vi "获取波形子集.vi"(1 "duration":dbl=1.0 caption="持续时间" format="%0.2f", 2 "start samples/time":dbl caption="起始采样/时间" format="%0.2f", 3 "时域波形图":waveform(dbl)[](graph)) -> (0 "时域波形图 2":waveform(dbl)[](graph))   [LabVIEW 2014]
uses:
  <vilib>/Waveform/WDTOps.llb/WDT Get Waveform Subset DBL.vi
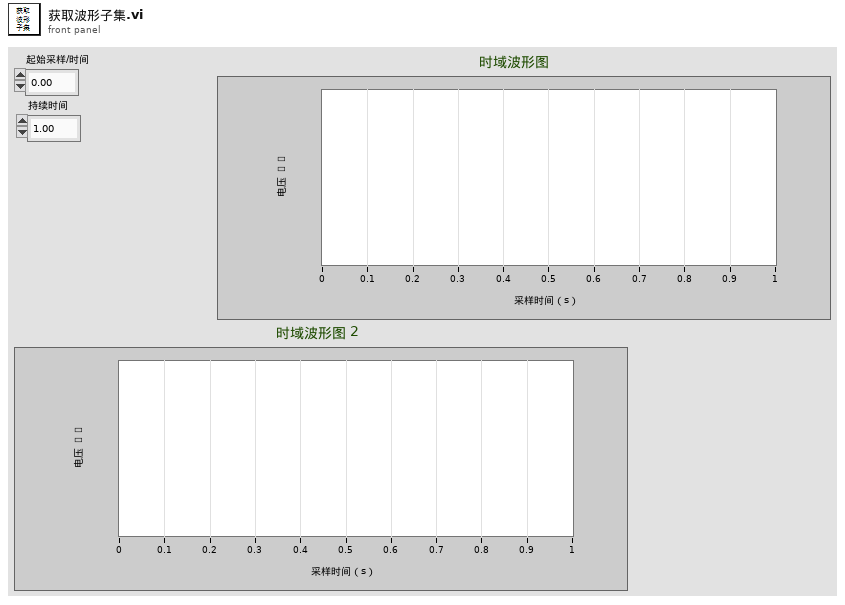
[diagram p1: front panel]
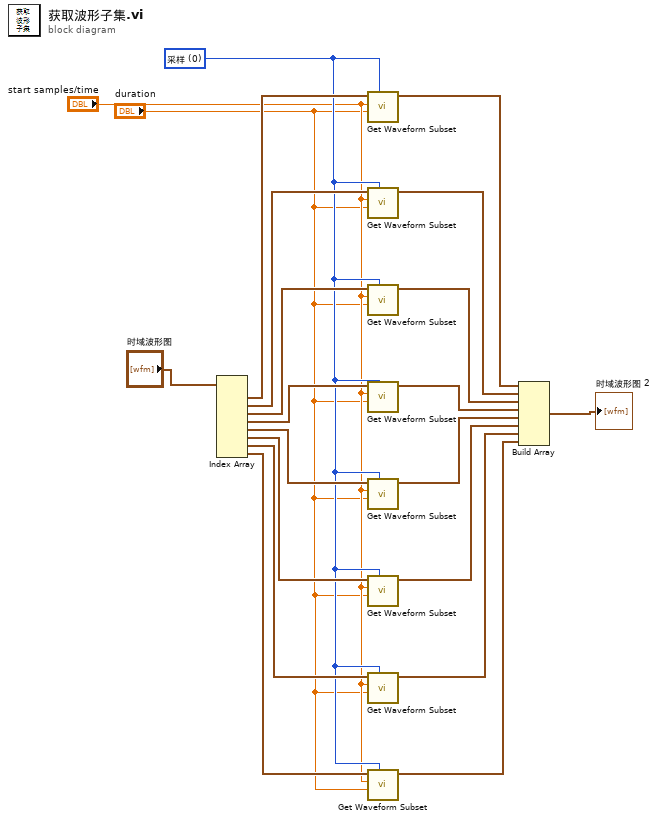
[diagram p0: block diagram]
diagram:
  w12 = u16 0 items=["采样", "相对时间"] ("start/duration format")
  n1 = Index Array(array="时域波形图") -> (element #1=w20:waveform(dbl), element #2=w19:waveform(dbl), element #3=w18:waveform(dbl), element #4=w17:waveform(dbl), element #5=w16:waveform(dbl), element #6=w15:waveform(dbl), element #7=w14:waveform(dbl), element #8=w13:waveform(dbl))  [unwired: 8 in]
  n2 = call-poly <vilib>:"Get Waveform Subset.vi"("start/duration format"=w12, "duration"="duration", "start samples/time"="start samples/time", "waveform in"=w20) -> ("waveform out"=w9:waveform(dbl))  [unwired: 2 in, 3 out]
  n3 = call-poly <vilib>:"Get Waveform Subset.vi"("start/duration format"=w12, "duration"="duration", "start samples/time"="start samples/time", "waveform in"=w19) -> ("waveform out"=w8:waveform(dbl))  [unwired: 2 in, 3 out]
  n4 = call-poly <vilib>:"Get Waveform Subset.vi"("start/duration format"=w12, "duration"="duration", "start samples/time"="start samples/time", "waveform in"=w18) -> ("waveform out"=w7:waveform(dbl))  [unwired: 2 in, 3 out]
  n5 = call-poly <vilib>:"Get Waveform Subset.vi"("start/duration format"=w12, "duration"="duration", "start samples/time"="start samples/time", "waveform in"=w17) -> ("waveform out"=w6:waveform(dbl))  [unwired: 2 in, 3 out]
  n6 = call-poly <vilib>:"Get Waveform Subset.vi"("start/duration format"=w12, "duration"="duration", "start samples/time"="start samples/time", "waveform in"=w16) -> ("waveform out"=w5:waveform(dbl))  [unwired: 2 in, 3 out]
  n7 = call-poly <vilib>:"Get Waveform Subset.vi"("start/duration format"=w12, "duration"="duration", "start samples/time"="start samples/time", "waveform in"=w15) -> ("waveform out"=w4:waveform(dbl))  [unwired: 2 in, 3 out]
  n8 = call-poly <vilib>:"Get Waveform Subset.vi"("start/duration format"=w12, "duration"="duration", "start samples/time"="start samples/time", "waveform in"=w14) -> ("waveform out"=w3:waveform(dbl))  [unwired: 2 in, 3 out]
  n9 = call-poly <vilib>:"Get Waveform Subset.vi"("start/duration format"=w12, "duration"="duration", "start samples/time"="start samples/time", "waveform in"=w13) -> ("waveform out"=w2:waveform(dbl))  [unwired: 2 in, 3 out]
  n10 = Build Array(w9, w8, w7, w6, w5, w4, w3, w2) -> (→"时域波形图 2":waveform(dbl)[])
